vi "Cal Plot Scale.vi"(8 "error in (no error)":errorcluster, 11 "Domain_Evolut_1D in":refnum<class "NI_Domain_Evolut_1D.lvclass">) -> (0 "error out":errorcluster, 1 "Y Scale":T1, 2 "X Scale":T1, 3 "Domain_Evolut_1D out":refnum<class "NI_Domain_Evolut_1D.lvclass">, 4 "# of t-points":i32)   [LabVIEW 2017, in "NI_PDE.lvlib" / "NI_Domain_Evolut_1D.lvclass"]
uses:
  <vilib>/gmath/pde.llb/DomainClass/Domain_Evolut_1D/NI_Domain_Evolut_1D.lvclass
  <vilib>/Utility/miscctls.llb/LVOffsetAndMultiplierTypeDef.ctl
  <vilib>/gmath/pde.llb/DomainClass/Domain_Evolut_1D/NI_Domain_Evolut_1D.lvclass/NI_Domain_Evolut_1D.ctl
  <vilib>/gmath/NI_PDE.lvlib
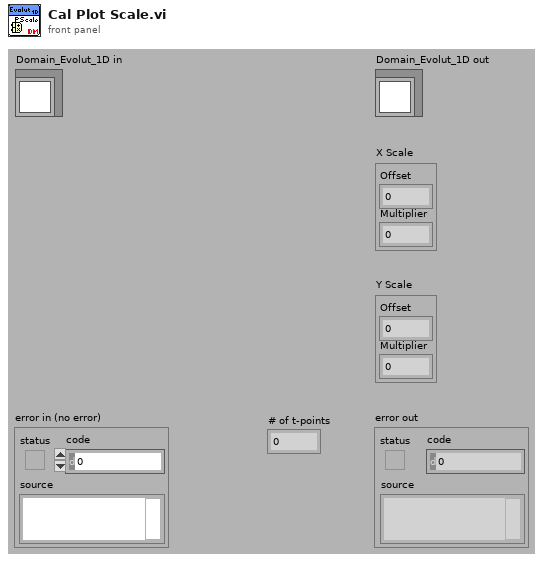
[diagram p1: front panel]
types:
  T1 = typedef "LVOffsetAndMultiplierTypeDef.ctl" = cluster{"Offset":dbl, "Multiplier":dbl}
  T2 = cluster{"initial t":dbl, "final t":dbl, "# of t-points":i32}
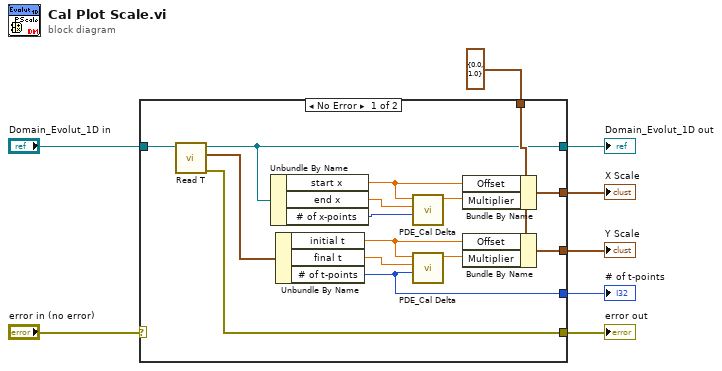
[diagram p0: block diagram]
diagram:
  n1 = case shown="No Error" "error in (no error)" {
    selector: "error in (no error)" -> [_ w26]
    tunnel: "Domain_Evolut_1D in" -> [w10 w25]
    tunnel: [w9 w25] -> w8
    tunnel: [w11 w26] -> w7
    tunnel: T1 {"Offset"=0.0, "Multiplier"=1.0} ("Offset and Multiplier") -> [w16 w24]
    tunnel: [w15 w24] -> w3
    tunnel: [w14 w24] -> w2
    tunnel: [w13 _] -> w1
    frame No Error {
      n2 = call-dynamic "Read T.vi"("Domain_Evolut.lvclass in"=w10) -> ("error out"=w11:errorcluster, "t"=w12:T2, "Domain_Evolut.lvclass out"=w9:refnum<class "NI_Domain_Evolut_1D.lvclass">)  [unwired: 1 in, 7 out]
      n3 = Unbundle By Name(w9) -> ("start x"=w22:dbl, "end x"=w20:dbl, "# of x-points"=w21:i32)
      n4 = Unbundle By Name(w12) -> ("initial t"=w18:dbl, "final t"=w19:dbl, "# of t-points"=w13:i32)
      n5 = call <vilib>:"PDE_Cal Delta.vi"("# of points"=w21, "end"=w20, "start"=w22) -> ("delta"=w23:dbl)  [unwired: 8 out]
      n6 = call <vilib>:"PDE_Cal Delta.vi"("# of points"=w13, "end"=w19, "start"=w18) -> ("delta"=w17:dbl)  [unwired: 8 out]
      n7 = Bundle By Name(cluster=w16, "Offset"=w22, "Multiplier"=w23) -> (w15:T1)
      n8 = Bundle By Name(cluster=w16, "Offset"=w18, "Multiplier"=w17) -> (w14:T1)
    }
    frame Error {
    }
  }
  "Domain_Evolut_1D out" <- w8
  "error out" <- w7
  "X Scale" <- w3
  "Y Scale" <- w2
  "# of t-points" <- w1
